vi "FGV_ArduinoCommsHandler.vi"(8 "Error In":errorcluster, 10 "Action":T1) -> (0 "error out":errorcluster)   [LabVIEW 2014]
uses:
  Typedef_ArduinoActions.ctl
  Typedef_FindPortActions.ctl
  Typedef_e2eArduinos.ctl
  Typedef_StepperCommand.ctl
  Typedef_GunSerial.ctl
  Typedef_Analyser1or2.ctl
  Typedef_AnalyserSerial.ctl
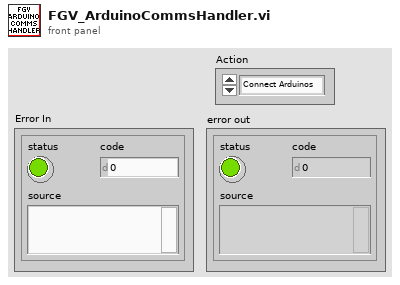
[diagram p1: front panel]
types:
  T1 = typedef "Typedef_ArduinoActions.ctl" = enum16{"Connect Arduinos", "Disconnect Arduinos"}
  T2 = typedef "Typedef_Analyser1or2.ctl" = enum16{"A1", "A2"}
  T3 = typedef "Typedef_AnalyserSerial.ctl" = enum16{"Connect", "RSE DAC", "RSE", "Lens", "Dx", "Dy", "Analyser Mean", "Inner Hemisphere", "Outer Hemisphere", "Get LENS", "Get DX", "Get DY", "Get All Set", "Get All Measured", "Lock FP", "Unlock FP", "ADC On", "ADC Off", "Read Response", "Disconnect"}
  T4 = typedef "Typedef_e2eArduinos.ctl" = enum16{"A1", "A2", "EG", "SC"}
  T5 = typedef "Typedef_FindPortActions.ctl" = enum16{"Reset List", "Find (e,2e) arduinos", "Get COM Port"}
  T6 = typedef "Typedef_GunSerial.ctl" = enum16{"Connect", "Coarse DAC", "Coarse Adjust", "Fine DAC", "Fine Adjust", "Get All Set", "Energy Adjust", "Grid", "Anode", "GL1B", "1DX", "1DY", "GL1C", "2DX", "2DY", "GL2B", "3DX", "3DY", "Read Response", "Disconnect"}
  T7 = typedef "Typedef_StepperCommand.ctl" = enum16{"Connect", "Disconnect", "Stop", "Get Voltage", "Get Angle", "Get Flags", "Get Status", "Set Angle", "Set Steps", "Set Max Rate", "Set Min Rate", "Set Acc. Rate", "Set Max Ang", "Set Max OP Ang", "Set Min Ang", "Set Crash Ang", "Set Hold Current", "Set Check Optos", "Set Check Ang Validity", "Read Response"}
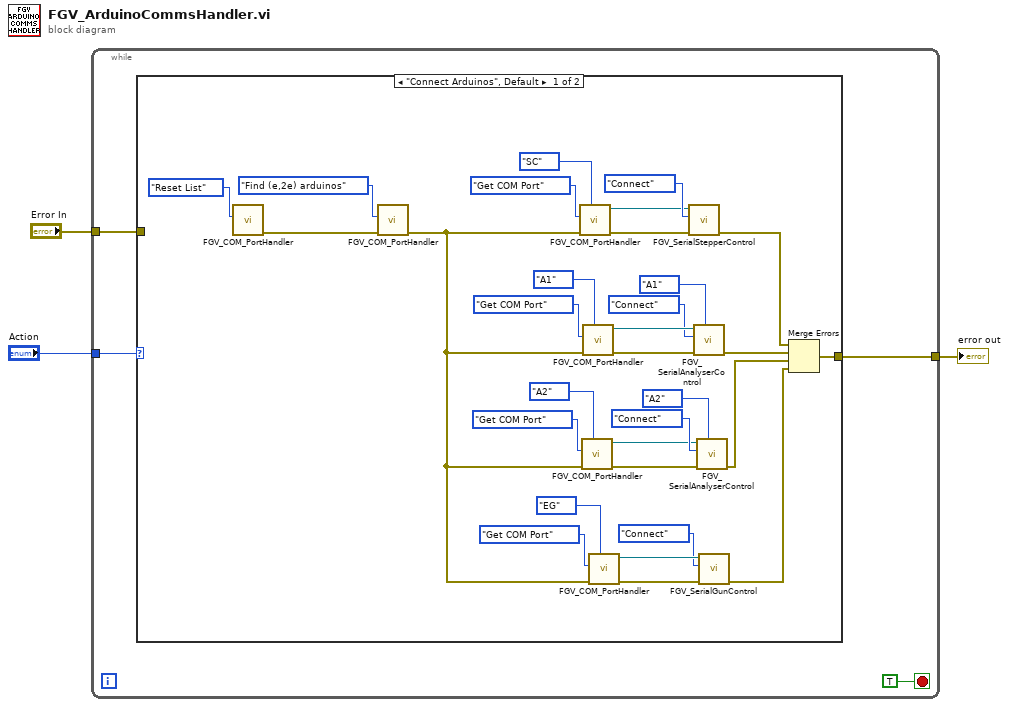
[diagram p0: block diagram]
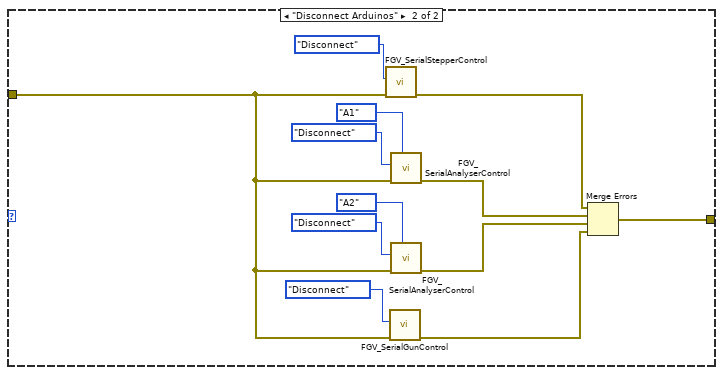
[diagram p2: hidden frame]
diagram:
  n1 = while {
    tunnel: [w6] -> w3
    tunnel: "Action" -> [w5]
    tunnel: "Error In" -> [w4]
    stop <- TRUE stop-if-true
    n2 = case shown="\"Connect Arduinos\", Default" w5 {
      tunnel: [w34 w49] -> w6
      tunnel: w4 -> [_ w39]
      frame "Connect Arduinos", Default {
        n3 = call "FGV_COM_PortHandler.vi"("Action"=Typedef_FindPortActions."Reset List") -> ("Error Out"=w13:errorcluster)  [unwired: 6 in, 1 out]
        n4 = call "FGV_COM_PortHandler.vi"("Error In"=w13, "Action"=Typedef_FindPortActions."Find (e,2e) arduinos") -> ("Error Out"=w33:errorcluster)  [unwired: 5 in, 1 out]
        n5 = call "FGV_COM_PortHandler.vi"("Device"=Typedef_e2eArduinos."SC", "Error In"=w33, "Action"=Typedef_FindPortActions."Get COM Port") -> ("Error Out"=w10:errorcluster, "COM Port"=w8:refnum<visa-resource-name>)  [unwired: 4 in]
        n6 = call "FGV_COM_PortHandler.vi"("Device"=Typedef_e2eArduinos."A2", "Error In"=w33, "Action"=Typedef_FindPortActions."Get COM Port") -> ("Error Out"=w16:errorcluster, "COM Port"=w17:refnum<visa-resource-name>)  [unwired: 4 in]
        n7 = call "FGV_COM_PortHandler.vi"("Device"=Typedef_e2eArduinos."A1", "Error In"=w33, "Action"=Typedef_FindPortActions."Get COM Port") -> ("Error Out"=w23:errorcluster, "COM Port"=w22:refnum<visa-resource-name>)  [unwired: 4 in]
        n8 = call "FGV_COM_PortHandler.vi"("Device"=Typedef_e2eArduinos."EG", "Error In"=w33, "Action"=Typedef_FindPortActions."Get COM Port") -> ("Error Out"=w29:errorcluster, "COM Port"=w30:refnum<visa-resource-name>)  [unwired: 4 in]
        n9 = call "FGV_SerialStepperControl.vi"("error in (no error)"=w10, "StepperCommand"=Typedef_StepperCommand."Connect", "VISA Refnum in"=w8) -> ("error out"=w35:errorcluster)  [unwired: 7 in, 1 out]
        n10 = call "FGV_SerialAnalyserControl.vi"("Analyser"=Typedef_Analyser1or2."A1", "error in (no error)"=w23, "Analyser Action"=Typedef_AnalyserSerial."Connect", "VISA Refnum in"=w22) -> ("error out"=w38:errorcluster)  [unwired: 6 in, 1 out]
        n11 = call "FGV_SerialAnalyserControl.vi"("Analyser"=Typedef_Analyser1or2."A2", "error in (no error)"=w16, "Analyser Action"=Typedef_AnalyserSerial."Connect", "VISA Refnum in"=w17) -> ("error out"=w37:errorcluster)  [unwired: 6 in, 1 out]
        n12 = call "FGV_SerialGunControl.vi"("error in (no error)"=w29, "Gun Action"=Typedef_GunSerial."Connect", "VISA Refnum in"=w30) -> ("error out"=w36:errorcluster)  [unwired: 6 in, 2 out]
        n13 = Merge Errors(w35, w38, w37, w36) -> (w34:errorcluster)
      }
      frame "Disconnect Arduinos" {
        n14 = call "FGV_SerialStepperControl.vi"("error in (no error)"=w39, "StepperCommand"=Typedef_StepperCommand."Disconnect") -> ("error out"=w42:errorcluster)  [unwired: 8 in, 1 out]
        n15 = call "FGV_SerialGunControl.vi"("error in (no error)"=w39, "Gun Action"=Typedef_GunSerial."Disconnect") -> ("error out"=w43:errorcluster)  [unwired: 7 in, 2 out]
        n16 = call "FGV_SerialAnalyserControl.vi"("Analyser"=Typedef_Analyser1or2."A1", "error in (no error)"=w39, "Analyser Action"=Typedef_AnalyserSerial."Disconnect") -> ("error out"=w41:errorcluster)  [unwired: 7 in, 1 out]
        n17 = call "FGV_SerialAnalyserControl.vi"("Analyser"=Typedef_Analyser1or2."A2", "error in (no error)"=w39, "Analyser Action"=Typedef_AnalyserSerial."Disconnect") -> ("error out"=w40:errorcluster)  [unwired: 7 in, 1 out]
        n18 = Merge Errors(w42, w41, w40, w43) -> (w49:errorcluster)
      }
    }
  }
  "error out" <- w3
